vi "GT_GetAxisPrfPos.vi"(10 "Axis in":T1=1 items=["Axis Control"=0, "Axis 1"=1, "Axis 2"=2, "Axis 3"=3, "Axis 4"=4, "Axis 5"=5, "Axis 6"=6, "Axis 7"=7, "Axis 8"=8, "Vector Space Control"=16, "Vector Space 1"=17, "Vector Space 2"=18, "Vector Space 3"=19, "Vector Space 4"=20], 11 "rtn_In":cluster{"rtn":i16, "Func":string}) -> (0 "Axis out":T1=1 items=["Axis Control"=0, "Axis 1"=1, "Axis 2"=2, "Axis 3"=3, "Axis 4"=4, "Axis 5"=5, "Axis 6"=6, "Axis 7"=7, "Axis 8"=8, "Vector Space Control"=16, "Vector Space 1"=17, "Vector Space 2"=18, "Vector Space 3"=19, "Vector Space 4"=20], 1 "count":i16, 2 "pValue":dbl, 3 "rtn_Out":cluster{"rtn":i16, "Func":string}, 4 "pClock":u32)   [LabVIEW 2014]
uses:
  <vilib>/Motion/FlexMotion/CustomControls/CustomControls.llb/AxisOrVectorSpaceControl To Control.flx
  VC6/gts.dll
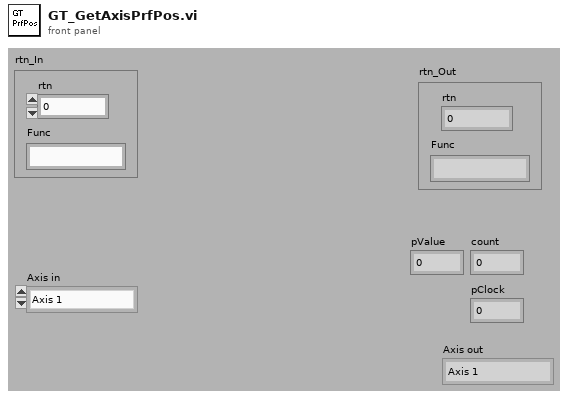
[diagram p1: front panel]
types:
  T1 = typedef "AxisOrVectorSpaceControl To Control.flx" = u16
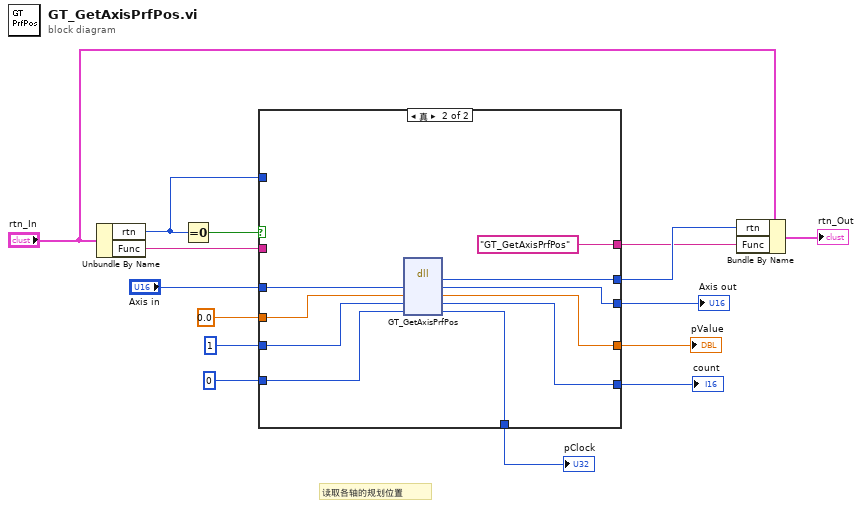
[diagram p0: block diagram]
diagram:
  # "读取各轴的规划位置"
  n1 = Unbundle By Name("rtn_In") -> ("rtn"=w6:i16, "Func"=w7:string)
  n2 = Equal To 0?(x=w6) -> (x = 0?=w15:bool)
  n3 = case shown="真" w15 {
    tunnel: "Axis in" -> [w19 w31]
    tunnel: 0.0 ("pValue") -> [w18 w30]
    tunnel: i16 1 ("count") -> [w17 w29]
    tunnel: u32 0 ("pClock") -> [w16 w28]
    tunnel: [w20 w27] -> w9
    tunnel: [w21 "GT_GetAxisPrfPos" ("Func")] -> w8
    tunnel: w7 -> [w21 _]
    tunnel: w6 -> [w20 _]
    tunnel: [w18 w25] -> w5
    tunnel: [w19 w24] -> w1
    tunnel: [w17 w23] -> w4
    tunnel: [w16 w22] -> w3
    frame False {
    }
    frame True {
      n4 = dll-call lib="PTH2Fabs DNewGTS AC-800LWin7版源程序-20170926gts85VC6gts.dll" fn="GT_GetAxisPrfPos"("axis"=w31, "pValue"=w30, "count"=w29, "pClock"=w28) -> ("rtn"=w27:i16, "axis"=w24:i16, "pValue"=w25:dbl, "count"=w23:i16, "pClock"=w22:u32)  [unwired: 3 in, 2 out]
    }
  }
  "pValue" <- w5
  "count" <- w4
  "pClock" <- w3
  "Axis out" <- w1
  n5 = Bundle By Name(cluster="rtn_In", "rtn"=w9, "Func"=w8) -> (→"rtn_Out":cluster{"rtn":i16, "Func":string})
